vi "sv_Check Expected Frequency.vi"(5 "frequency range":T1 {"stop frequency" format="%.2f"; "start frequency" format="%.2f"}, 7 "RBW":dbl format="%.2f", 11 "error in (no error)":errorcluster, 12 "expected fundamental frequency [Hz]":dbl format="%.2f") -> (14 "dup expected fundamental frequency [Hz]":dbl format="%.2f", 15 "error out":errorcluster)   [LabVIEW 2017, in "SoundVib_Distortion.lvlib"]
uses:
  <vilib>/addons/Sound and Vibration/svt_Distortion/SoundVib_Distortion.lvlib
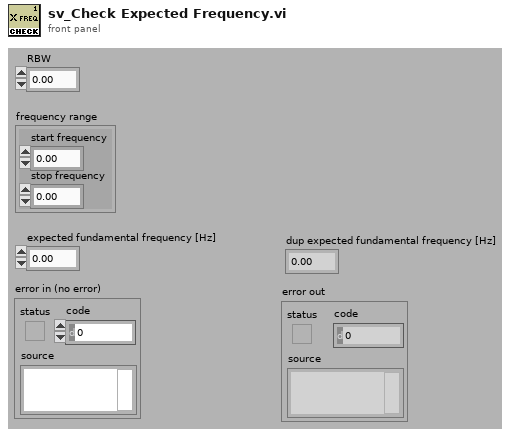
[diagram p1: front panel]
types:
  T1 = cluster{"start frequency":dbl, "stop frequency":dbl}
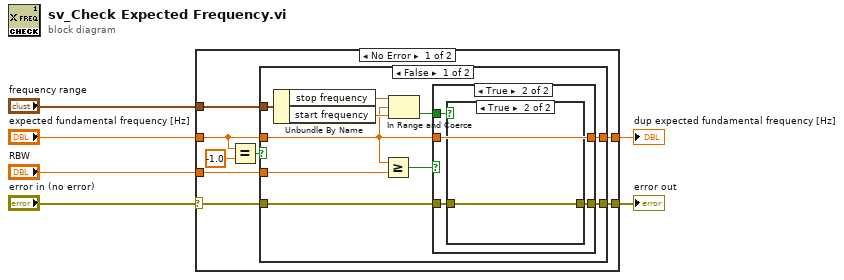
[diagram p0: block diagram]
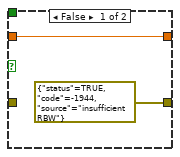
[diagram p2: hidden frame]
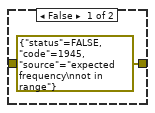
[diagram p3: hidden frame]
diagram:
  n1 = case shown="No Error" "error in (no error)" {
    selector: "error in (no error)" -> [w13 w36]
    tunnel: "expected fundamental frequency [Hz]" -> [w10 w35]
    tunnel: "frequency range" -> [w14 _]
    tunnel: [w12 w36] -> w4
    tunnel: [w8 w35] -> w5
    tunnel: "RBW" -> [w7 _]
    frame No Error {
      n2 = Equal?(x=w10, y=-1.0) -> (x = y?=w9:bool)
      n3 = case shown="False" w9 {
        tunnel: w14 -> [w24 _]
        tunnel: w13 -> [w23 w34]
        tunnel: [w22 w34] -> w12
        tunnel: w10 -> [w18 w33]
        tunnel: [w21 w33] -> w8
        tunnel: w7 -> [w17 _]
        frame False {
          n4 = Unbundle By Name(w24) -> ("stop frequency"=w20:dbl, "start frequency"=w19:dbl)
          n5 = Greater Or Equal?(x=w18, y=w17) -> (x >= y?=w16:bool)
          n6 = In Range and Coerce(upper limit=w20, x=w18, lower limit=w19) -> (In Range?=w15:bool)  [unwired: 1 out]
          n7 = case shown="True" w16 {
            tunnel: w23 -> [_ w27]
            tunnel: [errorcluster {"status"=TRUE, "code"=-1944, "source"="insufficient RBW"} ("error IO") w29] -> w22
            tunnel: w18 -> [w26 w30]
            tunnel: [w26 w30] -> w21
            tunnel: w15 -> [_ w28]
            frame False {
            }
            frame True {
              n8 = case shown="True" w28 {
                tunnel: [errorcluster {"status"=FALSE, "code"=1945, "source"="expected frequency\nnot in range"} ("error IO") w32] -> w29
                tunnel: w27 -> [_ w32]
                frame False {
                }
                frame True {
                }
              }
            }
          }
        }
        frame True {
        }
      }
    }
    frame Error {
    }
  }
  "dup expected fundamental frequency [Hz]" <- w5
  "error out" <- w4
